vi "Timeout.vi"(8 "error in (no error)":errorcluster, 11 "BluelinesRedlines in":refnum<class "BluelinesRedlines.lvclass">) -> (0 "error out":errorcluster, 3 "BluelinesRedlines out":refnum<class "BluelinesRedlines.lvclass">)   [LabVIEW 2020, in "VolatusGUIElements.lvlib" / "BluelinesRedlines.lvclass"]
uses:
  BluelinesRedlines.lvclass
  C:/dev/lv20CE/relink/lv-volatus/VolatusGUI/GUI Element/GUI Element.lvclass
  BLRL Control.ctl
  BluelinesRedlines.lvclass/BluelinesRedlines.ctl
  VolatusGUI/GUI Element/GUI Element.lvclass/GUI Element.ctl
  VolatusGUI/BluelinesRedlines Source/BluelinesRedlines Source.lvclass
  VolatusGUI/GUI Element/GUI Element.lvclass
  VolatusGUI/BluelinesRedlines Source/BLRL Type.ctl
  C:/dev/lv20CE/relink/lv-volatus/VolatusGUIElements/BluelinesRedlines/BluelinesRedlines.lvclass
  C:/dev/lv20CE/relink/lv-volatus/VolatusGUI/OnValueChangeHandler/OnValueChangeHandler.lvclass
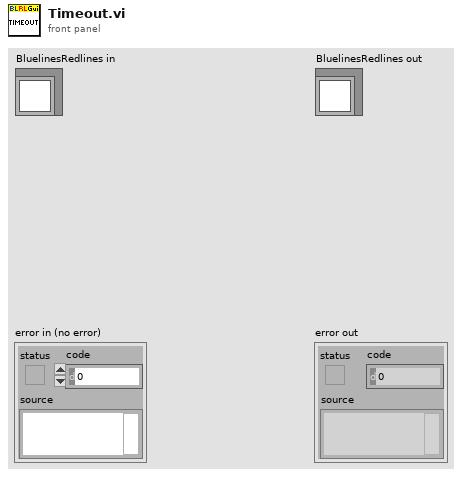
[diagram p1: front panel]
types:
  T1 = typedef "VolatusGUIElements.lvlib/BluelinesRedlines.lvclass/BLRL Control.ctl" = cluster{"Blue Lines":cluster{"Channel":string, "Low":string, "Value":dbl, "High":string, "Color":u32, "Remove Channel":bool}[], "Red Lines":cluster{"Channel":string, "Low":string, "Value":dbl, "High":string, "Color":u32, "Remove Channel":bool}[], "Import":bool, "Export":bool, "Blueline Status":bool, "Redlines Status":bool, "Group":string, "New Group":bool, "Dup Group":bool, "Remove Group":bool, "Add Blue Channel":bool, "Add Red Channel":bool, "Reset Redlines":bool}
  T2 = typedef "VolatusGUIElements.lvlib/BluelinesRedlines.lvclass/Channel Info.ctl" = cluster{"Channel":refnum<class "Channel DBL.lvclass">, "Redline":bool}
  T3 = map{string, refnum<class "BluelinesRedlines Source.lvclass">}
  T4 = typedef "VolatusGUI.lvlib/BluelinesRedlines Source.lvclass/BLRL Type.ctl" = enum16{"Blueline", "Redline"}
  T5 = cluster{"Channel":string, "Low":string, "Value":dbl, "High":string, "Color":u32, "Remove Channel":bool}
  T6 = typedef "VolatusGUI.lvlib/BluelinesRedlines Source.lvclass/BLRL Config.ctl" = cluster{"Bluelines":T7[], "Redlines":T7[]}
  T7 = typedef "VolatusGUI.lvlib/BluelinesRedlines Source.lvclass/Range Limit Config.ctl" = cluster{"Channel":string, "Low Limit":dbl, "High Limit":dbl}
  T8 = cluster{cluster{"Channel":string, "Low":string, "Value":dbl, "High":string, "Color":u32, "Remove Channel":bool}[], bool[]}
  T9 = cluster{"Channel":string, "Low":string, "Value":dbl, "High":string, "Color":u32, "Remove Channel":bool}[]
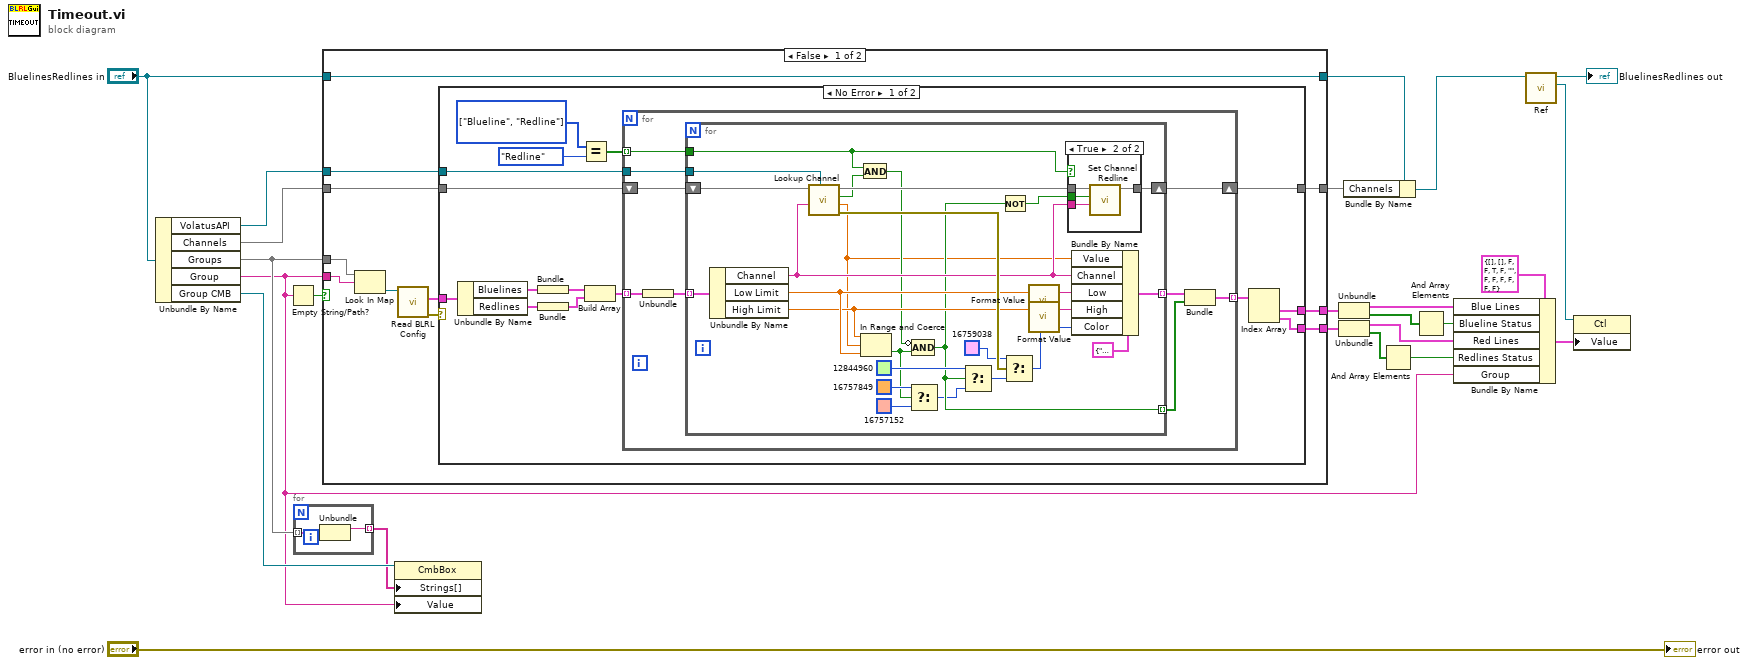
[diagram p0: block diagram]
diagram:
  n1 = Unbundle By Name("BluelinesRedlines in") -> ("VolatusAPI"=w8:refnum<class "VolatusAPI.lvclass">, "Channels"=w9:map{string, T2}, "Groups"=w5:T3, "Group"=w2:string, "Group CMB"=w4:refnum<vi>)
  n2 = Empty String/Path?(string/path=w2) -> (empty?=w23:bool)
  n3 = for {
    tunnel: w5 -> [w26] mode=indexing
    tunnel: [w25] -> w3 mode=indexing
    n4 = Unbundle(w26) -> ("Name"=w25:string)  [unwired: 1 out]
  }
  n5 = case shown="False" w23 {
    tunnel: w2 -> [w37 _]
    tunnel: "BluelinesRedlines in" -> [w33 w96]
    tunnel: [w33 w96] -> w21
    tunnel: [w32 _] -> w20
    tunnel: [w31 _] -> w19
    tunnel: w9 -> [w30 w95]
    tunnel: w5 -> [w29 _]
    tunnel: w8 -> [w28 _]
    tunnel: [w27 w95] -> w6
    frame False {
      n6 = Look In Map(map=w29, key=w37) -> (value=w36:refnum<class "BluelinesRedlines Source.lvclass">)  [unwired: 1 in, 1 out]
      n7 = call-dynamic "Read BLRL Config.vi"("BluelinesRedlines Source in"=w36) -> ("error out"=w34:errorcluster, "BLRL Config"=w35:T6)  [unwired: 8 in, 1 out]
      n8 = case shown="No Error" w34 {
        tunnel: w35 -> [w52 _]
        tunnel: w30 -> [w47 w94]
        tunnel: w28 -> [w46 _]
        tunnel: [w43 _] -> w32
        tunnel: [w42 _] -> w31
        tunnel: [w41 w94] -> w27
        frame No Error {
          w40 = T4[] [enum."Blueline", enum."Redline"] items=["Blueline", "Redline"]
          n9 = Unbundle By Name(w52) -> ("Bluelines"=w51:T7[], "Redlines"=w50:T7[])
          n10 = Bundle("Bluelines"=w51) -> (w49:cluster{"Bluelines":T7[]})  [unwired: 1 in]
          n11 = Bundle("Redlines"=w50) -> (w48:cluster{"Redlines":T7[]})  [unwired: 1 in]
          n12 = Equal?(x=w40, y=BLRL_Type."Redline" ("BLRL Type")) -> (x = y?=w38:bool[])
          n13 = Build Array(w49, w48) -> (w45:cluster{"Redlines":T7[]}[])
          n14 = for {
            shift-right: [w57] -> w41
            shift-left: w47 -> [w60]
            tunnel: w46 -> [w59]
            tunnel: w45 -> [w61] mode=indexing
            tunnel: [w55] -> w44 mode=indexing
            tunnel: w38 -> [w53] mode=indexing
            n15 = Unbundle(w61) -> ("Redlines"=w58:T7[])
            n16 = for {
              shift-right: [w72] -> w57
              shift-left: w60 -> [w86]
              tunnel: w59 -> [w85]
              tunnel: w58 -> [w87] mode=indexing
              tunnel: [w79] -> w56 mode=indexing
              tunnel: [w70] -> w54 mode=indexing
              tunnel: w53 -> [w62]
              n17 = Unbundle By Name(w87) -> ("Channel"=w71:string, "Low Limit"=w77:dbl, "High Limit"=w75:dbl)
              n18 = call "Lookup Channel.vi"("VolatusAPI"=w85, "Name"=w71, "Channels in"=w86) -> ("error out"=w88:errorcluster, "Value"=w63:dbl, "Redline"=w73:bool, "Channels"=w84:map{string, T2})  [unwired: 5 in]
              n19 = And(x=w62, y=w73) -> (x .and. y?=w64:bool)
              n20 = In Range and Coerce(upper limit=w75, x=w63, lower limit=w77) -> (In Range?=w66:bool)  [unwired: 1 out]
              n21 = Select(t=u32 16757849, s=w66, f=u32 16757152) -> (s? t:f=w65:u32)
              n22 = Compound Arithmetic op=AND(invert w64, w66) -> (w70:bool)
              n23 = Select(t=u32 12844960, s=w70, f=w65) -> (s? t:f=w82:u32)
              n24 = Not(x=w70) -> (.not. x?=w69:bool)
              n25 = Select(t=u32 16759038, s=w88, f=w82) -> (s? t:f=w80:u32)
              n26 = call "Format Value.vi"("Value"=w77) -> ("String"=w76:string)  [unwired: 6 in]
              n27 = call "Format Value.vi"("Value"=w75) -> ("String"=w74:string)  [unwired: 6 in]
              n28 = case shown="True" w62 {
                tunnel: w84 -> [w89 w93]
                tunnel: [w89 w92] -> w72
                tunnel: w71 -> [_ w91]
                tunnel: w69 -> [_ w90]
                frame False {
                }
                frame True {
                  n29 = call "Set Channel Redline.vi"("Name"=w91, "Redline"=w90, "Channels in"=w93) -> ("Channels"=w92:map{string, T2})  [unwired: 7 in, 1 out]
                }
              }
              n30 = Bundle By Name(cluster=T5 {"Channel"="", "Low"="", "Value"=0.0, "High"="", "Color"=0, "Remove Channel"=FALSE} ("Channel Range"), "Value"=w63, "Channel"=w71, "Low"=w76, "High"=w74, "Color"=w80) -> (w79:T5)
            }
            n31 = Bundle(w56, w54) -> (w55:T8)  [unwired: 1 in]
          }
          n32 = Index Array(array=w44) -> (element #1=w43:T8, element #2=w42:T8)  [unwired: 2 in]
        }
        frame Error {
        }
      }
    }
    frame True {
    }
  }
  n33 = property class="CmbBox"(reference=w4, "Strings[]"=w3, "Value"=w2) -> ()  [unwired: 1 in, 2 out]
  n34 = Unbundle(w20) -> (w1:T9, w14:bool[])
  n35 = Unbundle(w19) -> (w15:T9, w17:bool[])
  n36 = Bundle By Name(cluster=w21, "Channels"=w6) -> (w7:refnum<class "BluelinesRedlines.lvclass">)
  n37 = And Array Elements(Boolean array=w17) -> (logical AND=w16:bool)
  n38 = And Array Elements(Boolean array=w14) -> (logical AND=w13:bool)
  n39 = Bundle By Name(cluster=T1 {"Blue Lines"=[], "Red Lines"=[], "Import"=FALSE, "Export"=FALSE, "Blueline Status"=TRUE, "Redlines Status"=FALSE, "Group"="", "New Group"=FALSE, "Dup Group"=FALSE, "Remove Group"=FALSE, "Add Blue Channel"=FALSE, "Add Red Channel"=FALSE, "Reset Redlines"=FALSE} ("RedlinesBluelines"), "Blue Lines"=w1, "Blueline Status"=w13, "Red Lines"=w15, "Redlines Status"=w16, "Group"=w2) -> (w10:T1)
  n40 = call "Ref.vi"("GUI Element in"=w7) -> ("Ref"=w11:refnum<vi>, "GUI Element out"=→"BluelinesRedlines out":refnum<class "BluelinesRedlines.lvclass">)  [unwired: 9 in]
  n41 = property class="Ctl"(reference=w11, "Value"=w10) -> ()  [unwired: 1 in, 2 out]
  "error out" <- "error in (no error)"
